vi "Load Category Instruments.vi"(8 "error in (no error)":errorcluster, 11 "Category in":refnum<class "Category.lvclass">) -> (0 "error out":errorcluster, 3 "Category out":refnum<class "Category.lvclass">)   [LabVIEW 2015, in "Category Library.lvlib" / "Category.lvclass"]
uses:
  Category.lvclass
  Category.lvclass/Category.ctl
  Instrument Information/Instrument.lvclass
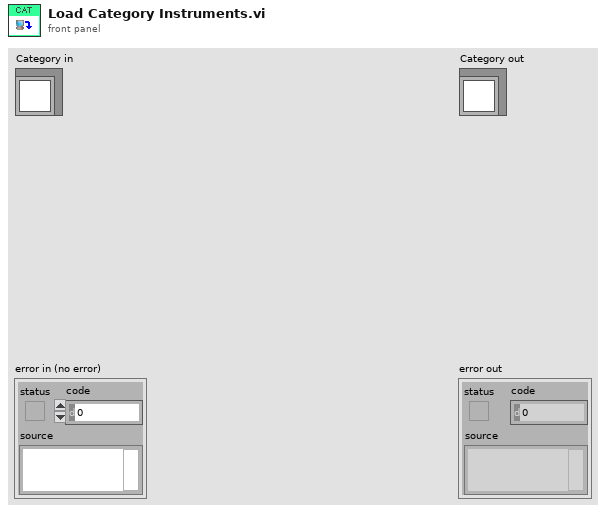
[diagram p1: front panel]
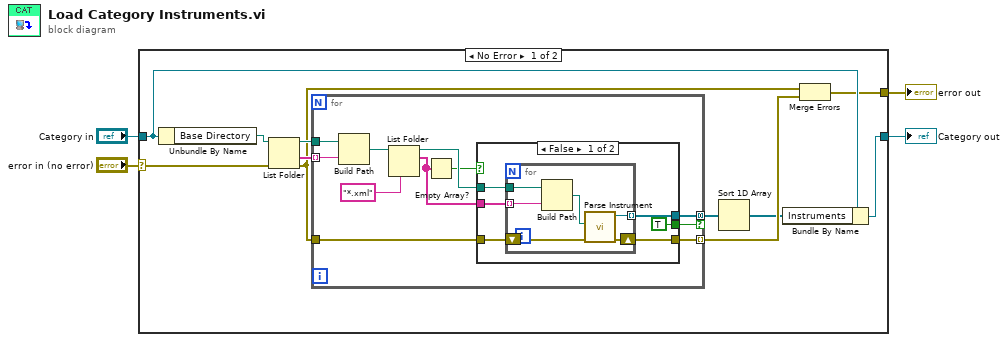
[diagram p0: block diagram]
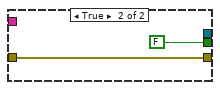
[diagram p2: hidden frame]
diagram:
  n1 = case shown="No Error" "error in (no error)" {
    selector: "error in (no error)" -> [w10 w42]
    tunnel: [w7 w42] -> w3
    tunnel: [w11 w41] -> w1
    tunnel: "Category in" -> [w12 w41]
    frame No Error {
      n2 = Unbundle By Name(w12) -> ("Base Directory"=w15:path)
      n3 = List Folder(path=w15, error in=w10) -> (path out=w13:path, folder names=w14:string[], error out=w9:errorcluster)  [unwired: 2 in, 1 out]
      n4 = for {
        tunnel: w13 -> [w26]
        tunnel: w14 -> [w25] mode=indexing
        tunnel: [w24] -> w6 mode=concatenating if=w16
        tunnel: w9 -> [w23]
        tunnel: [w22] -> w8 mode=indexing
        n5 = Build Path(base path=w26, name or relative path=w25) -> (appended path=w20:path)
        n6 = List Folder(path=w20, pattern="*.xml") -> (path out=w19:path, filenames=w18:string[])  [unwired: 2 in, 2 out]
        n7 = Empty Array?(array=w18) -> (empty?=w17:bool)
        n8 = case shown="False" w17 {
          tunnel: [w32 _] -> w24
          tunnel: w23 -> [w31 w39]
          tunnel: [w30 w39] -> w22
          tunnel: w19 -> [w29 _]
          tunnel: w18 -> [w27 _]
          tunnel: [TRUE FALSE] -> w16
          frame False {
            n9 = for {
              tunnel: [w38] -> w32 mode=indexing
              tunnel: w29 -> [w35]
              shift-right: [w36] -> w30
              shift-left: w31 -> [w37]
              tunnel: w27 -> [w33] mode=indexing
              n10 = Build Path(base path=w35, name or relative path=w33) -> (appended path=w34:path)
              n11 = call "Parse Instrument.vi"("error in (no error)"=w37, "path to XML document"=w34) -> ("error out"=w36:errorcluster, "Instrument"=w38:refnum<class "Instrument.lvclass">)  [unwired: 8 in]
            }
          }
          frame True {
          }
        }
      }
      n12 = Sort 1D Array(array=w6) -> (sorted array=w5:refnum<class "Instrument.lvclass">[])
      n13 = Bundle By Name(cluster=w12, "Instruments"=w5) -> (w11:refnum<class "Category.lvclass">)
      n14 = Merge Errors(w9, w8) -> (w7:errorcluster)
    }
    frame Error {
    }
  }
  "error out" <- w3
  "Category out" <- w1
